vi "Read Data Bus.vi"(8 "error in (no error)":errorcluster, 11 "IO in":refnum<class "IO.lvclass">) -> (0 "error out":errorcluster, 3 "IO out":refnum<class "IO.lvclass">)   [LabVIEW 2021, in "IO.lvclass"]
uses:
  IO.lvclass
  IO.lvclass/IO.ctl
  <vilib>/DAQmx/read.llb/DAQmx Read (Digital 1D Bool NChan 1Samp 1Line).vi
  <vilib>/DAQmx/miscellaneous.llb/DAQmx Fill In Error Info.vi
  <resource>/objmgr/daqmx.rc
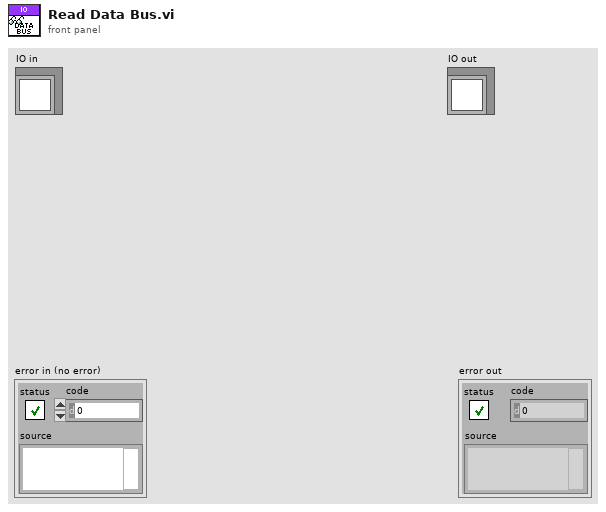
[diagram p1: front panel]
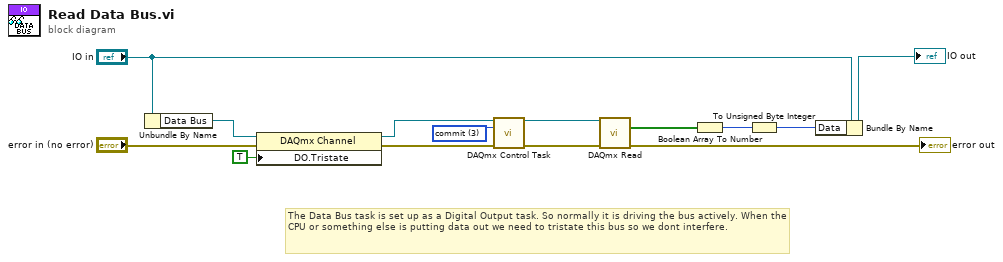
[diagram p0: block diagram]
diagram:
  w1 = 3 items=["verify"=2, "reserve"=4, "commit"=3, "unreserve"=5, "abort"=6] ("action")
  # "The Data Bus task is set up as a Digital Output task. So normally it is driving the bus actively. When the CPU or something else is putting data out we need to tristate this bus so we dont interfere."
  n1 = Unbundle By Name("IO in") -> ("Data Bus"=w12:refnum<k21>)
  n2 = property class="DAQmx Channel"(reference=w12, error in="error in (no error)", "DO.Tristate"=TRUE) -> (reference out=w6:refnum<k21>, error out=w3:errorcluster)
  n3 = call <vilib>:"DAQmx Control Task.vi"("task/channels in"=w6, "action"=w1, "error in"=w3) -> ("task out"=w5:refnum<k21>, "error out"=w2:errorcluster)  [unwired: 11 in]
  n4 = call-poly <vilib>:"DAQmx Read.vi"("task/channels in"=w5, "error in"=w2) -> ("data"=w14:bool[], "error out"=→"error out":errorcluster)  [unwired: 11 in, 1 out]
  n5 = Boolean Array To Number(Boolean array=w14) -> (number=w11:u32)
  n6 = To Unsigned Byte Integer(number=w11) -> (unsigned 8bit integer=w8:u8)
  n7 = Bundle By Name(cluster="IO in", "Data"=w8) -> (→"IO out":refnum<class "IO.lvclass">)
